vi "Write Element of Sections.vi"(8 "error in (no error)":errorcluster, 9 "Section":refnum<class "Section.lvclass">, 10 "index":i32, 11 "Configuration in":refnum<class "Configuration.lvclass">) -> (0 "error out":errorcluster, 3 "Configuration out":refnum<class "Configuration.lvclass">)   [LabVIEW 2015, in "Configuration.lvlib" / "Configuration.lvclass"]
doc: "Write section by index to class private data."
uses:
  Configuration.lvclass
  Section/Section.lvclass
  Configuration.lvclass/Configuration.ctl
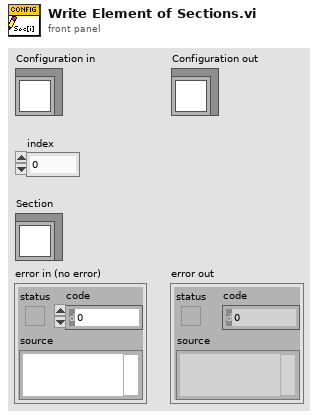
[diagram p1: front panel]
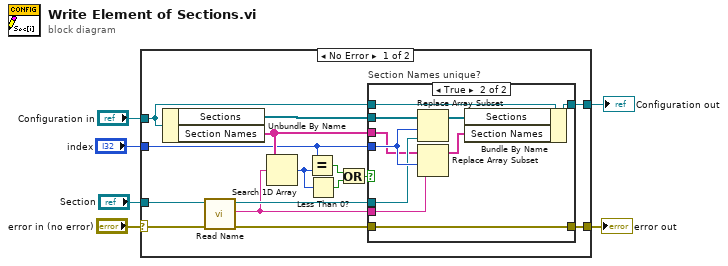
[diagram p0: block diagram]
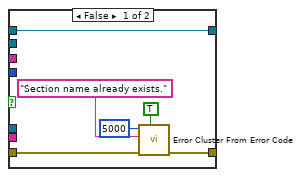
[diagram p2: hidden frame]
diagram:
  n1 = case shown="No Error" "error in (no error)" {
    selector: "error in (no error)" -> [w16 w38]
    tunnel: [w12 w38] -> w5
    tunnel: [w21 w39] -> w3
    tunnel: "Configuration in" -> [w20 w39]
    tunnel: "Section" -> [w18 _]
    tunnel: "index" -> [w11 _]
    frame No Error {
      n2 = Unbundle By Name(w20) -> ("Sections"=w19:refnum<class "Section.lvclass">[], "Section Names"=w15:string[])
      n3 = call "Read Name.vi"("error in (no error)"=w16, "Section in"=w18) -> ("error out"=w13:errorcluster, "Name"=w14:string, "Section out"=w17:refnum<class "Section.lvclass">)  [unwired: 7 in]
      n4 = Search 1D Array(1D array=w15, element=w14) -> (index of element=w10:i32)  [unwired: 1 in]
      n5 = Equal?(x=w11, y=w10) -> (x = y?=w9:bool)
      n6 = Less Than 0?(x=w10) -> (x < 0?=w8:bool)
      n7 = Or(x=w9, y=w8) -> (x .or. y?=w7:bool)
      n8 = case "Section Names unique?" shown="True" w7 {
        tunnel: [w27 w37] -> w21
        tunnel: w20 -> [w27 w36]
        tunnel: w19 -> [_ w35]
        tunnel: w11 -> [_ w33]
        tunnel: w17 -> [_ w32]
        tunnel: w15 -> [_ w30]
        tunnel: w14 -> [_ w29]
        tunnel: w13 -> [w26 w28]
        tunnel: [w25 w28] -> w12
        frame False {
          n9 = call <vilib>:"Error Cluster From Error Code.vi"("show call chain? (False)"=TRUE, "error in (no error)"=w26, "error message (\"\")"="Section name already exists." ("error message (\"\")"), "error code (0)"=5000) -> ("error out"=w25:errorcluster)  [unwired: 5 in]
        }
        frame True {
          n10 = Replace Array Subset(array=w35, new element=w32, index=w33) -> (w34:refnum<class "Section.lvclass">[])
          n11 = Replace Array Subset(array=w30, new element=w29, index=w33) -> (w31:string[])
          n12 = Bundle By Name(cluster=w36, "Sections"=w34, "Section Names"=w31) -> (w37:refnum<class "Configuration.lvclass">)
        }
      }
    }
    frame Error {
    }
  }
  "error out" <- w5
  "Configuration out" <- w3
